vi "Render Section.vi"(8 "Error In":errorcluster, 10 "Section":refnum<class "Section.lvclass">, 11 "Renderer In":refnum<class "Renderer.lvclass">) -> (0 "Error Out":errorcluster, 2 "Output":string, 3 "Renderer Out":refnum<class "Renderer.lvclass">)   [LabVIEW 2018, in "Toolkit.lvlib" / "Renderer.lvclass"]
uses:
  Renderer.lvclass
  Nodes/Section/Section.lvclass
  Nodes/Section/Section.lvclass/Section.ctl
  Data/Array/Array.lvclass
  Data/Array/Array.lvclass/Array.ctl
  Renderer.lvclass/Renderer.ctl
  Data/Boolean/Boolean.lvclass
  Data/Function/Function.lvclass
  Data/String/String.lvclass
  Data/String/String.lvclass/String.ctl
  Data/Path/Path.lvclass
  Data/Path/Path.lvclass/Path.ctl
  Data/Datum/Datum.lvclass
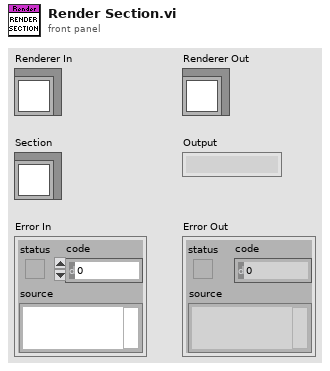
[diagram p1: front panel]
types:
  T1 = typedef "Toolkit.lvlib/Data.lvlib/Types.ctl" = enum16{"Array", "Boolean", "Function", "Map", "Null", "Pair", "Path", "String", "Unknown"}
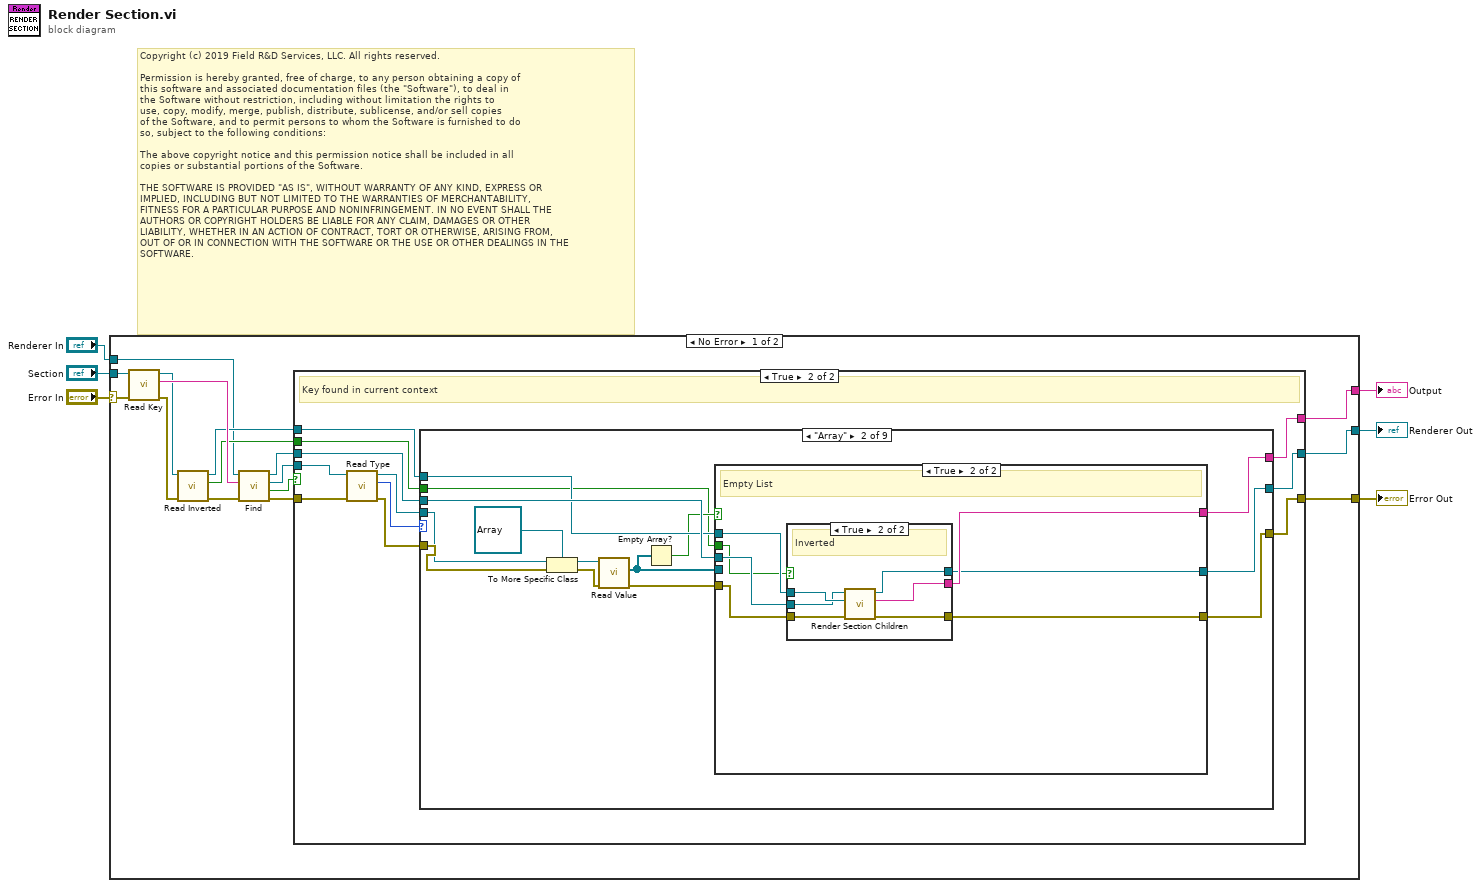
[diagram p0: block diagram]
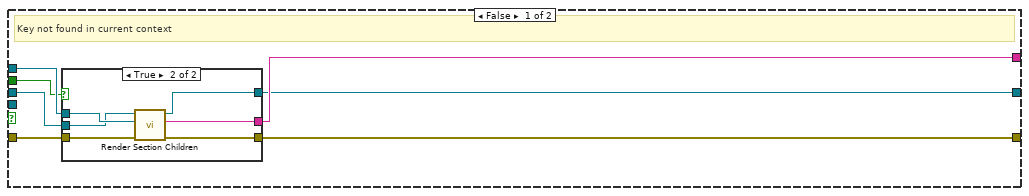
[diagram p2: hidden frame]
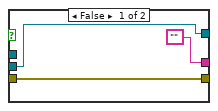
[diagram p3: hidden frame]
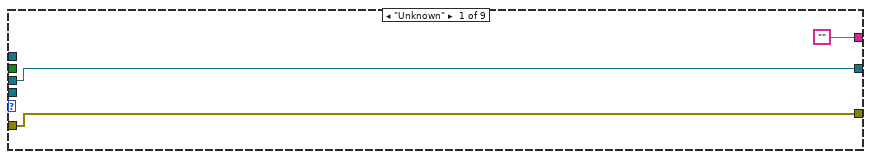
[diagram p4: hidden frame]
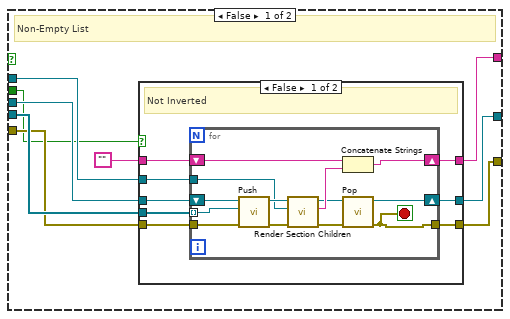
[diagram p5: hidden frame]
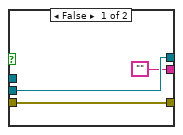
[diagram p7: hidden frame]
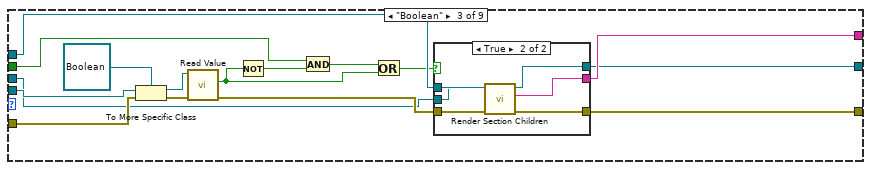
[diagram p8: hidden frame]
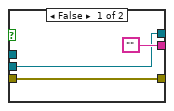
[diagram p9: hidden frame]
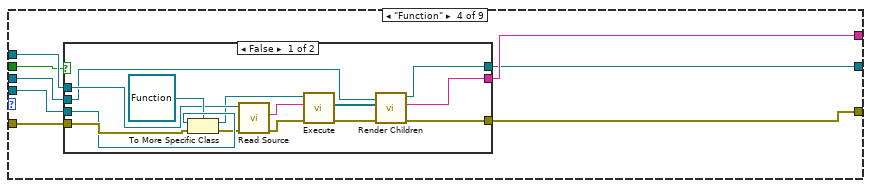
[diagram p10: hidden frame]
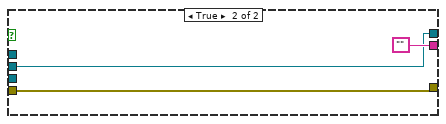
[diagram p11: hidden frame]
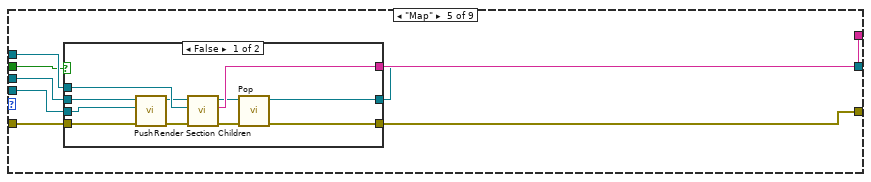
[diagram p12: hidden frame]
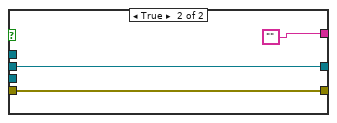
[diagram p13: hidden frame]
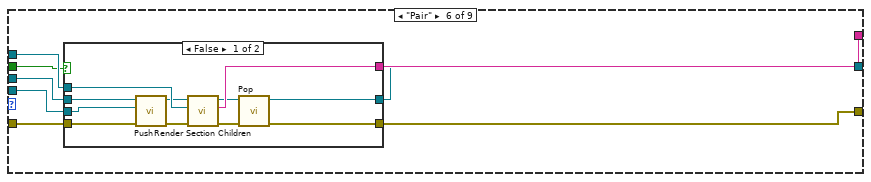
[diagram p14: hidden frame]
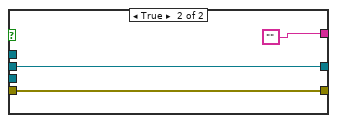
[diagram p15: hidden frame]
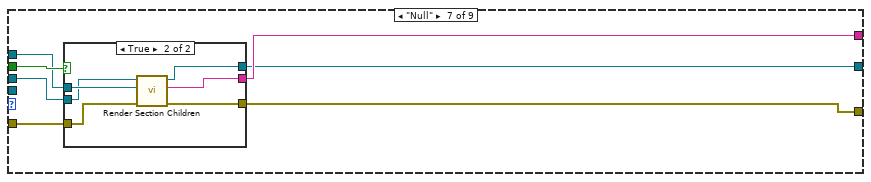
[diagram p16: hidden frame]
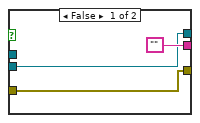
[diagram p17: hidden frame]
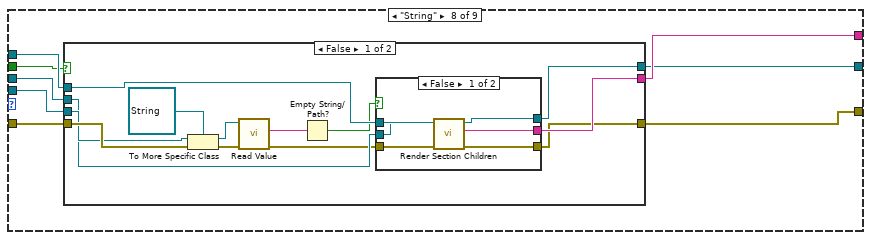
[diagram p18: hidden frame]
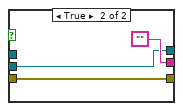
[diagram p19: hidden frame]
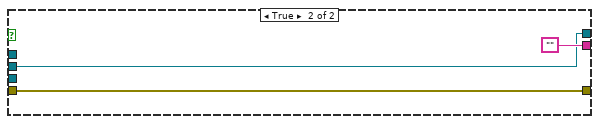
[diagram p20: hidden frame]
diagram:
  # "Copyright (c) 2019 Field R&D Services, LLC. All rights reserved.\n\nPermission is hereby granted, free of charge, to any person obtaining a copy of\nthis software and associated documentation files (the \"Software\"), to deal in\nthe Software without restriction, including without limitation the rights to\nuse, copy, modify, merge, publish, distribute, sublicense, and/or sell copies\nof the Software, and to permit persons to whom the Software is furnished to do\nso, subject to the following conditions:\n\nThe above copyright notice and this permission notice shall be included in all\ncopies or substantial portions of the Software.\n\nTHE SOFTWARE IS PROVIDED \"AS IS\", WITHOUT WARRANTY OF ANY KIND, EXPRESS OR\nIMPLIED, INCLUDING BUT NOT LIMITED TO THE WARRANTIES OF MERCHANTABILITY,\nFITNESS FOR A PARTICULAR PURPOSE AND NONINFRINGEMENT. IN NO EVENT SHALL THE\nAUTHORS OR COPYRIGHT HOLDERS BE LIABLE FOR ANY CLAIM, DAMAGES OR OTHER\nLIABILITY, WHETHER IN AN ACTION OF CONTRACT, TORT OR OTHERWISE, ARISING FROM,\nOUT OF OR IN CONNECTION WITH THE SOFTWARE OR THE USE OR OTHER DEALINGS IN THE\nSOFTWARE."
  n1 = case shown="No Error" "Error In" {
    selector: "Error In" -> [w10 w296]
    tunnel: "Section" -> [w11 _]
    tunnel: [w7 w296] -> w5
    tunnel: [w8 ""] -> w4
    tunnel: "Renderer In" -> [w12 w294]
    tunnel: [w9 w294] -> w1
    frame No Error {
      n2 = call "Read Key.vi"("Error In"=w10, "Section In"=w11) -> ("Error Out"=w15:errorcluster, "Key"=w18:string, "Section Out"=w17:refnum<class "Section.lvclass">)  [unwired: 7 in]
      n3 = call "Read Inverted.vi"("Error In"=w15, "Section In"=w17) -> ("Error Out"=w14:errorcluster, "Inverted"=w13:bool, "Section Out"=w16:refnum<class "Section.lvclass">)  [unwired: 7 in]
      n4 = call "Find.vi"("Error In"=w14, "Key"=w18, "Renderer In"=w12) -> ("Error Out"=w21:errorcluster, "Found?"=w22:bool, "Datum"=w20:refnum<class "Datum.lvclass">, "Renderer Out"=w19:refnum<class "Renderer.lvclass">)  [unwired: 5 in]
      n5 = case shown="True" w22 {
        tunnel: [w24 w49] -> w8
        tunnel: [w28 w48] -> w7
        tunnel: w21 -> [w29 w40]
        tunnel: w20 -> [_ w47]
        tunnel: w16 -> [w27 w46]
        tunnel: w19 -> [w25 w45]
        tunnel: w13 -> [w26 w44]
        tunnel: [w23 w43] -> w9
        frame False {
          # "Key not found in current context"
          n6 = case shown="True" w26 {
            tunnel: w29 -> [w31 w38]
            tunnel: [w31 w37] -> w28
            tunnel: w27 -> [_ w36]
            tunnel: ["" w35] -> w24
            tunnel: w25 -> [w30 w33]
            tunnel: [w30 w34] -> w23
            frame False {
            }
            frame True {
              n7 = call "Render Section Children.vi"("Error In"=w38, "Section"=w36, "Renderer In"=w33) -> ("Error Out"=w37:errorcluster, "Output"=w35:string, "Renderer Out"=w34:refnum<class "Renderer.lvclass">)  [unwired: 6 in]
            }
          }
        }
        frame True {
          # "Key found in current context"
          n8 = call-dynamic "Read Type.vi"("Error In"=w40, "Datum In"=w47) -> ("Error Out"=w39:errorcluster, "Type"=w41:T1, "Datum Out"=w42:refnum<class "Datum.lvclass">)  [unwired: 7 in]
          n9 = case shown="\"Array\"" w41 {
            tunnel: w39 -> [w52 w66 w131 w148 w169 w191 w215 w233 w266]
            tunnel: ["" w58 w126 w144 w168 w190 w212 w231 w264] -> w49
            tunnel: [w52 w59 w125 w145 w172 w194 w214 w230 w263] -> w48
            tunnel: w42 -> [_ w65 w130 w147 w170 w192 _ w232 w265]
            tunnel: w46 -> [_ w57 w124 w143 w171 w193 w213 w229 w262]
            tunnel: w45 -> [w50 w61 w123 w146 w173 w195 w211 w228 w261]
            tunnel: w44 -> [_ w53 w119 w142 w167 w189 w216 w227 w260]
            tunnel: [w50 w55 w117 w141 w166 w188 w210 w226 w259] -> w43
            frame "Unknown" {
            }
            frame "Array" {
              n10 = To More Specific Class(target class=refnum<class "Array.lvclass"> refnum ("Toolkit.lvlib:Data.lvlib:Array.lvclass"), reference=w65, error in=w66) -> (specific class reference=w63:refnum<class "Array.lvclass">, error out=w62:errorcluster)
              n11 = call "Read Value.vi"("Error In"=w62, "Array In"=w63) -> ("Error Out"=w60:errorcluster, "Value"=w56:refnum<class "Datum.lvclass">[])  [unwired: 7 in, 1 out]
              n12 = Empty Array?(array=w56) -> (empty?=w54:bool)
              n13 = case shown="True" w54 {
                tunnel: w56 -> [w75 _]
                tunnel: w61 -> [w74 w102]
                tunnel: w60 -> [w73 w104]
                tunnel: [w72 w103] -> w59
                tunnel: [w71 w105] -> w58
                tunnel: w57 -> [w69 w106]
                tunnel: [w70 w101] -> w55
                tunnel: w53 -> [w68 w100]
                frame False {
                  # "Non-Empty List"
                  n14 = case shown="False" w68 {
                    tunnel: w75 -> [w83 _]
                    tunnel: w74 -> [w82 w98]
                    tunnel: w73 -> [w81 w97]
                    tunnel: [w80 w97] -> w72
                    tunnel: [w79 w99] -> w71
                    tunnel: [w78 w98] -> w70
                    tunnel: w69 -> [w77 _]
                    tunnel: "" -> [w76 w99]
                    frame False {
                      # "Not Inverted"
                      n15 = for {
                        tunnel: w83 -> [w95] mode=indexing
                        tunnel: w81 -> [w96]
                        shift-right: [w94] -> w78
                        shift-left: w82 -> [w85]
                        tunnel: [w86] -> w80
                        shift-right: [w92] -> w79
                        shift-left: w76 -> [w93]
                        tunnel: w77 -> [w87]
                        stop <- w86 stop-if-true
                        n16 = call "Push.vi"("Error In"=w96, "Datum"=w95, "Renderer In"=w85) -> ("Error Out"=w90:errorcluster, "Renderer Out"=w91:refnum<class "Renderer.lvclass">)  [unwired: 7 in]
                        n17 = call "Render Section Children.vi"("Error In"=w90, "Section"=w87, "Renderer In"=w91) -> ("Error Out"=w89:errorcluster, "Output"=w88:string, "Renderer Out"=w84:refnum<class "Renderer.lvclass">)  [unwired: 6 in]
                        n18 = Concatenate Strings(w93, w88) -> (w92:string)
                        n19 = call "Pop.vi"("Error In"=w89, "Renderer In"=w84) -> ("Error Out"=w86:errorcluster, "Renderer Out"=w94:refnum<class "Renderer.lvclass">)  [unwired: 7 in, 1 out]
                      }
                    }
                    frame True {
                      # "Inverted"
                    }
                  }
                }
                frame True {
                  # "Empty List"
                  n20 = case shown="True" w100 {
                    tunnel: w106 -> [_ w115]
                    tunnel: ["" w114] -> w105
                    tunnel: w104 -> [w108 w111]
                    tunnel: [w108 w113] -> w103
                    tunnel: w102 -> [w109 w110]
                    tunnel: [w109 w112] -> w101
                    frame False {
                    }
                    frame True {
                      # "Inverted"
                      n21 = call "Render Section Children.vi"("Error In"=w111, "Section"=w115, "Renderer In"=w110) -> ("Error Out"=w113:errorcluster, "Output"=w114:string, "Renderer Out"=w112:refnum<class "Renderer.lvclass">)  [unwired: 6 in]
                    }
                  }
                }
              }
            }
            frame "Boolean" {
              n22 = To More Specific Class(target class=refnum<class "Boolean.lvclass"> refnum ("Toolkit.lvlib:Data.lvlib:Boolean.lvclass"), reference=w130, error in=w131) -> (specific class reference=w116:refnum<class "Boolean.lvclass">, error out=w128:errorcluster)
              n23 = call "Read Value.vi"("Error In"=w128, "Boolean In"=w116) -> ("Error Out"=w127:errorcluster, "Value"=w122:bool)  [unwired: 7 in, 1 out]
              n24 = Not(x=w122) -> (.not. x?=w121:bool)
              n25 = And(x=w119, y=w121) -> (x .and. y?=w120:bool)
              n26 = Or(x=w120, y=w122) -> (x .or. y?=w118:bool)
              n27 = case shown="True" w118 {
                tunnel: w127 -> [w133 w140]
                tunnel: ["" w137] -> w126
                tunnel: [w133 w138] -> w125
                tunnel: w124 -> [_ w139]
                tunnel: w123 -> [w132 w135]
                tunnel: [w132 w136] -> w117
                frame False {
                }
                frame True {
                  n28 = call "Render Section Children.vi"("Error In"=w140, "Section"=w139, "Renderer In"=w135) -> ("Error Out"=w138:errorcluster, "Output"=w137:string, "Renderer Out"=w136:refnum<class "Renderer.lvclass">)  [unwired: 6 in]
                }
              }
            }
            frame "Function" {
              n29 = case shown="False" w142 {
                tunnel: w148 -> [w162 w165]
                tunnel: w147 -> [w161 _]
                tunnel: w146 -> [w151 w163]
                tunnel: [w158 w165] -> w145
                tunnel: [w157 ""] -> w144
                tunnel: w143 -> [w156 _]
                tunnel: [w150 w163] -> w141
                frame False {
                  n30 = To More Specific Class(target class=refnum<class "Function.lvclass"> refnum ("Toolkit.lvlib:Data.lvlib:Function.lvclass"), reference=w161, error in=w162) -> (specific class reference=w149:refnum<class "Function.lvclass">, error out=w154:errorcluster)
                  n31 = call-dynamic "Read Source.vi"("Error In"=w154, "Node In"=w156) -> ("Error Out"=w153:errorcluster, "Source"=w152:string)  [unwired: 7 in, 1 out]
                  n32 = call-dynamic "Execute.vi"("Error In"=w153, "Source"=w152, "Function In"=w149) -> ("Error Out"=w155:errorcluster, "Nodes"=w159:refnum<class "Node.lvclass">[])  [unwired: 6 in, 1 out]
                  n33 = call "Render Children.vi"("Error In"=w155, "Children"=w159, "Renderer In"=w151) -> ("Error Out"=w158:errorcluster, "Output"=w157:string, "Renderer Out"=w150:refnum<class "Renderer.lvclass">)  [unwired: 6 in]
                }
                frame True {
                }
              }
            }
            frame "Map" {
              n34 = case shown="False" w167 {
                tunnel: w173 -> [w175 w185]
                tunnel: [w184 w187] -> w172
                tunnel: w171 -> [w183 _]
                tunnel: w170 -> [w179 _]
                tunnel: w169 -> [w178 w187]
                tunnel: [w177 ""] -> w168
                tunnel: [w176 w185] -> w166
                frame False {
                  n35 = call "Push.vi"("Error In"=w178, "Datum"=w179, "Renderer In"=w175) -> ("Error Out"=w181:errorcluster, "Renderer Out"=w182:refnum<class "Renderer.lvclass">)  [unwired: 7 in]
                  n36 = call "Render Section Children.vi"("Error In"=w181, "Section"=w183, "Renderer In"=w182) -> ("Error Out"=w180:errorcluster, "Output"=w177:string, "Renderer Out"=w174:refnum<class "Renderer.lvclass">)  [unwired: 6 in]
                  n37 = call "Pop.vi"("Error In"=w180, "Renderer In"=w174) -> ("Error Out"=w184:errorcluster, "Renderer Out"=w176:refnum<class "Renderer.lvclass">)  [unwired: 7 in, 1 out]
                }
                frame True {
                }
              }
            }
            frame "Pair" {
              n38 = case shown="False" w189 {
                tunnel: w195 -> [w197 w207]
                tunnel: [w206 w209] -> w194
                tunnel: w193 -> [w205 _]
                tunnel: w192 -> [w201 _]
                tunnel: w191 -> [w200 w209]
                tunnel: [w199 ""] -> w190
                tunnel: [w198 w207] -> w188
                frame False {
                  n39 = call "Push.vi"("Error In"=w200, "Datum"=w201, "Renderer In"=w197) -> ("Error Out"=w203:errorcluster, "Renderer Out"=w204:refnum<class "Renderer.lvclass">)  [unwired: 7 in]
                  n40 = call "Render Section Children.vi"("Error In"=w203, "Section"=w205, "Renderer In"=w204) -> ("Error Out"=w202:errorcluster, "Output"=w199:string, "Renderer Out"=w196:refnum<class "Renderer.lvclass">)  [unwired: 6 in]
                  n41 = call "Pop.vi"("Error In"=w202, "Renderer In"=w196) -> ("Error Out"=w206:errorcluster, "Renderer Out"=w198:refnum<class "Renderer.lvclass">)  [unwired: 7 in, 1 out]
                }
                frame True {
                }
              }
            }
            frame "Null" {
              n42 = case shown="True" w216 {
                tunnel: w215 -> [w218 w225]
                tunnel: [w218 w224] -> w214
                tunnel: w213 -> [_ w223]
                tunnel: ["" w222] -> w212
                tunnel: w211 -> [w217 w220]
                tunnel: [w217 w221] -> w210
                frame False {
                }
                frame True {
                  n43 = call "Render Section Children.vi"("Error In"=w225, "Section"=w223, "Renderer In"=w220) -> ("Error Out"=w224:errorcluster, "Output"=w222:string, "Renderer Out"=w221:refnum<class "Renderer.lvclass">)  [unwired: 6 in]
                }
              }
            }
            frame "String" {
              n44 = case shown="False" w227 {
                tunnel: w233 -> [w246 w258]
                tunnel: w232 -> [w245 _]
                tunnel: [w244 ""] -> w231
                tunnel: [w243 w258] -> w230
                tunnel: w229 -> [w242 _]
                tunnel: w228 -> [w241 w256]
                tunnel: [w234 w256] -> w226
                frame False {
                  n45 = To More Specific Class(target class=refnum<class "String.lvclass"> refnum ("Toolkit.lvlib:Data.lvlib:String.lvclass"), reference=w245, error in=w246) -> (specific class reference=w238:refnum<class "String.lvclass">, error out=w239:errorcluster)
                  n46 = call "Read Value.vi"("Error In"=w239, "String In"=w238) -> ("Error Out"=w235:errorcluster, "Value"=w237:string)  [unwired: 7 in, 1 out]
                  n47 = Empty String/Path?(string/path=w237) -> (empty?=w236:bool)
                  n48 = case shown="False" w236 {
                    tunnel: [w250 ""] -> w244
                    tunnel: [w251 w254] -> w243
                    tunnel: w242 -> [w252 _]
                    tunnel: w241 -> [w247 w253]
                    tunnel: w235 -> [w249 w254]
                    tunnel: [w248 w253] -> w234
                    frame False {
                      n49 = call "Render Section Children.vi"("Error In"=w249, "Section"=w252, "Renderer In"=w247) -> ("Error Out"=w251:errorcluster, "Output"=w250:string, "Renderer Out"=w248:refnum<class "Renderer.lvclass">)  [unwired: 6 in]
                    }
                    frame True {
                    }
                  }
                }
                frame True {
                }
              }
            }
            frame "Path" {
              n50 = case shown="False" w260 {
                tunnel: w266 -> [w281 w293]
                tunnel: w265 -> [w280 _]
                tunnel: [w279 ""] -> w264
                tunnel: [w278 w293] -> w263
                tunnel: w262 -> [w277 _]
                tunnel: w261 -> [w276 w291]
                tunnel: [w272 w291] -> w259
                frame False {
                  n51 = To More Specific Class(target class=refnum<class "Path.lvclass"> refnum ("Toolkit.lvlib:Data.lvlib:Path.lvclass"), reference=w280, error in=w281) -> (specific class reference=w274:refnum<class "Path.lvclass">, error out=w275:errorcluster)
                  n52 = call "Read Value.vi"("Error In"=w275, "Path In"=w274) -> ("Error Out"=w273:errorcluster, "Value"=w268:path)  [unwired: 7 in, 1 out]
                  n53 = Not A Number/Path/Refnum?(number/path/refnum=w268) -> (NaN/Path/Refnum?=w269:bool)
                  n54 = Empty String/Path?(string/path=w268) -> (empty?=w270:bool)
                  n55 = Compound Arithmetic op=OR(w269, w270) -> (invert w267:bool)
                  n56 = case shown="True" w267 {
                    tunnel: ["" w288] -> w279
                    tunnel: [w283 w289] -> w278
                    tunnel: w277 -> [_ w290]
                    tunnel: w276 -> [w282 w285]
                    tunnel: w273 -> [w283 w287]
                    tunnel: [w282 w286] -> w272
                    frame False {
                    }
                    frame True {
                      n57 = call "Render Section Children.vi"("Error In"=w287, "Section"=w290, "Renderer In"=w285) -> ("Error Out"=w289:errorcluster, "Output"=w288:string, "Renderer Out"=w286:refnum<class "Renderer.lvclass">)  [unwired: 6 in]
                    }
                  }
                }
                frame True {
                }
              }
            }
          }
        }
      }
    }
    frame Error {
    }
  }
  "Error Out" <- w5
  "Output" <- w4
  "Renderer Out" <- w1
